vi "Main_Sigma_Single Scan_3.vi"() -> ()   [LabVIEW 2012]
uses:
  <vilib>/DAQmx/read.llb/DAQmx Read (Analog 1D DBL 1Chan NSamp).vi
  <vilib>/Instr/_visa.llb/VISA Configure Serial Port (Instr).vi
  <vilib>/DAQmx/create/channels.llb/DAQmx Create Channel (AI-Voltage-Basic).vi
  <vilib>/DAQmx/configure/timing.llb/DAQmx Timing (Sample Clock).vi
  <vilib>/DAQmx/configure/trigger.llb/DAQmx Start Trigger (Digital Edge).vi
  <vilib>/DAQmx/miscellaneous.llb/DAQmx Fill In Error Info.vi
  Global_data.vi
  <resource>/objmgr/daqmx.rc
  <vilib>/Platform/NI_3dgraph.lvlib
panel:
  out "Start. Pos.Y":dbl=18.8 format="%#.4f"
  out "숫자형 2":i32
  out "Start Pos. X":dbl=-22.5 format="%#.4f"
  out "숫자형":i32
  out "x < 0?":bool
  out "열거형":T1(ring)
  in  "Direction (+)":bool=TRUE
  out "No. X":i32=249
  out "No. Y":i32=13
  in  "X-length":dbl=5.0
  in  "Step X":dbl=0.02
  in  "COM Port":refnum<visa-resource-name>="COM1"
  in  "Baud Rate":u32=9600
  in  "Data bits":u16=8 min=5 max=8 step=1
  in  "stop bits":u16(ring)=10 items=["1.0"=10, "1.5"=15, "2.0"=20]
  in  "Parity":u16(ring) items=["None", "Odd", "Even", "Mark", "Space"]
  in  "1 Min":dbl=0.4
  in  "2 Max":dbl=4.0
  in  "1  Max":dbl=4.0
  in  "2 Min":dbl=0.4
  in  "Y-length":dbl=10.0
  in  "Step Y":dbl=0.1
  in  "1 Rate":dbl=0.2
  in  "2 Rate":dbl=0.4
  in  "Travel per Pulse (mm)":dbl=0.002
  in  "Cur. Pos X":dbl=-22.5 format="%#.4f"
  in  "Cur. Pos Y":dbl=18.8 format="%#.4f"
  in  "Save Speed":bool
  out "Move X":bool
  in  "Physical Channel":tag="Dev1/ai1"
  in  "Min Voltage":dbl=-0.2
  in  "Max Voltage":dbl=0.2
  in  "Terminal Configuration":i32(ring)=10083 items=["default"=-1, "RSE"=10083, "NRSE"=10078, "Differential"=10106, "Pseudodifferential"=12529]
  in  "rate":dbl=450000.0 format="%0.2f"
  in  "samples per channel":i32=100
  in  "3D Surface":refnum<k7>(container)
  in  "Stop Scan 3":bool
  in  "X-length count":dbl=20.0
  out "No.data":i32=3250
  in  "Save Scan mode":bool caption="Save Process"
  in  "Plot style":i32(ring)=5 items=["cwLine"=1, "cwPoint"=2, "cwLinePoint"=3, "cwHiddenLine"=4, "cwSurface"=5, "cwSurfaceLine"=6, "cwSurfaceNormal"=7, "cwContourLine"=8, "cwSurfaceContour"=9]
  in  "ViewMode":i32(ring) items=["cwViewXYPlane", "cwViewXZPlane", "cwViewYZPlane", "cwViewUserDefined"]
  in  "Emergency Stop":bool
  in  "Stop 3":bool
  in  "Home Y":bool
  in  "Home X":bool
  in  "Back":bool
  in  "Front":bool
  in  "Left":bool
  in  "Right":bool
  in  "Stop Scan":bool
  in  "Move Distance (mm)":dbl=5.0
  in  "Scan":bool
  in  "Open":bool
  in  "Edge":i32(ring)=10280 items=["Rising"=10280, "Falling"=10171]
  in  "Digital Trigger Source":tag="/Dev1/PFI8"
  # "Sensor  Channel"
  # "COM  Setting"
  # "Trigger Settings"
  # "Speed  Setting"
  # "Scan  Setting"
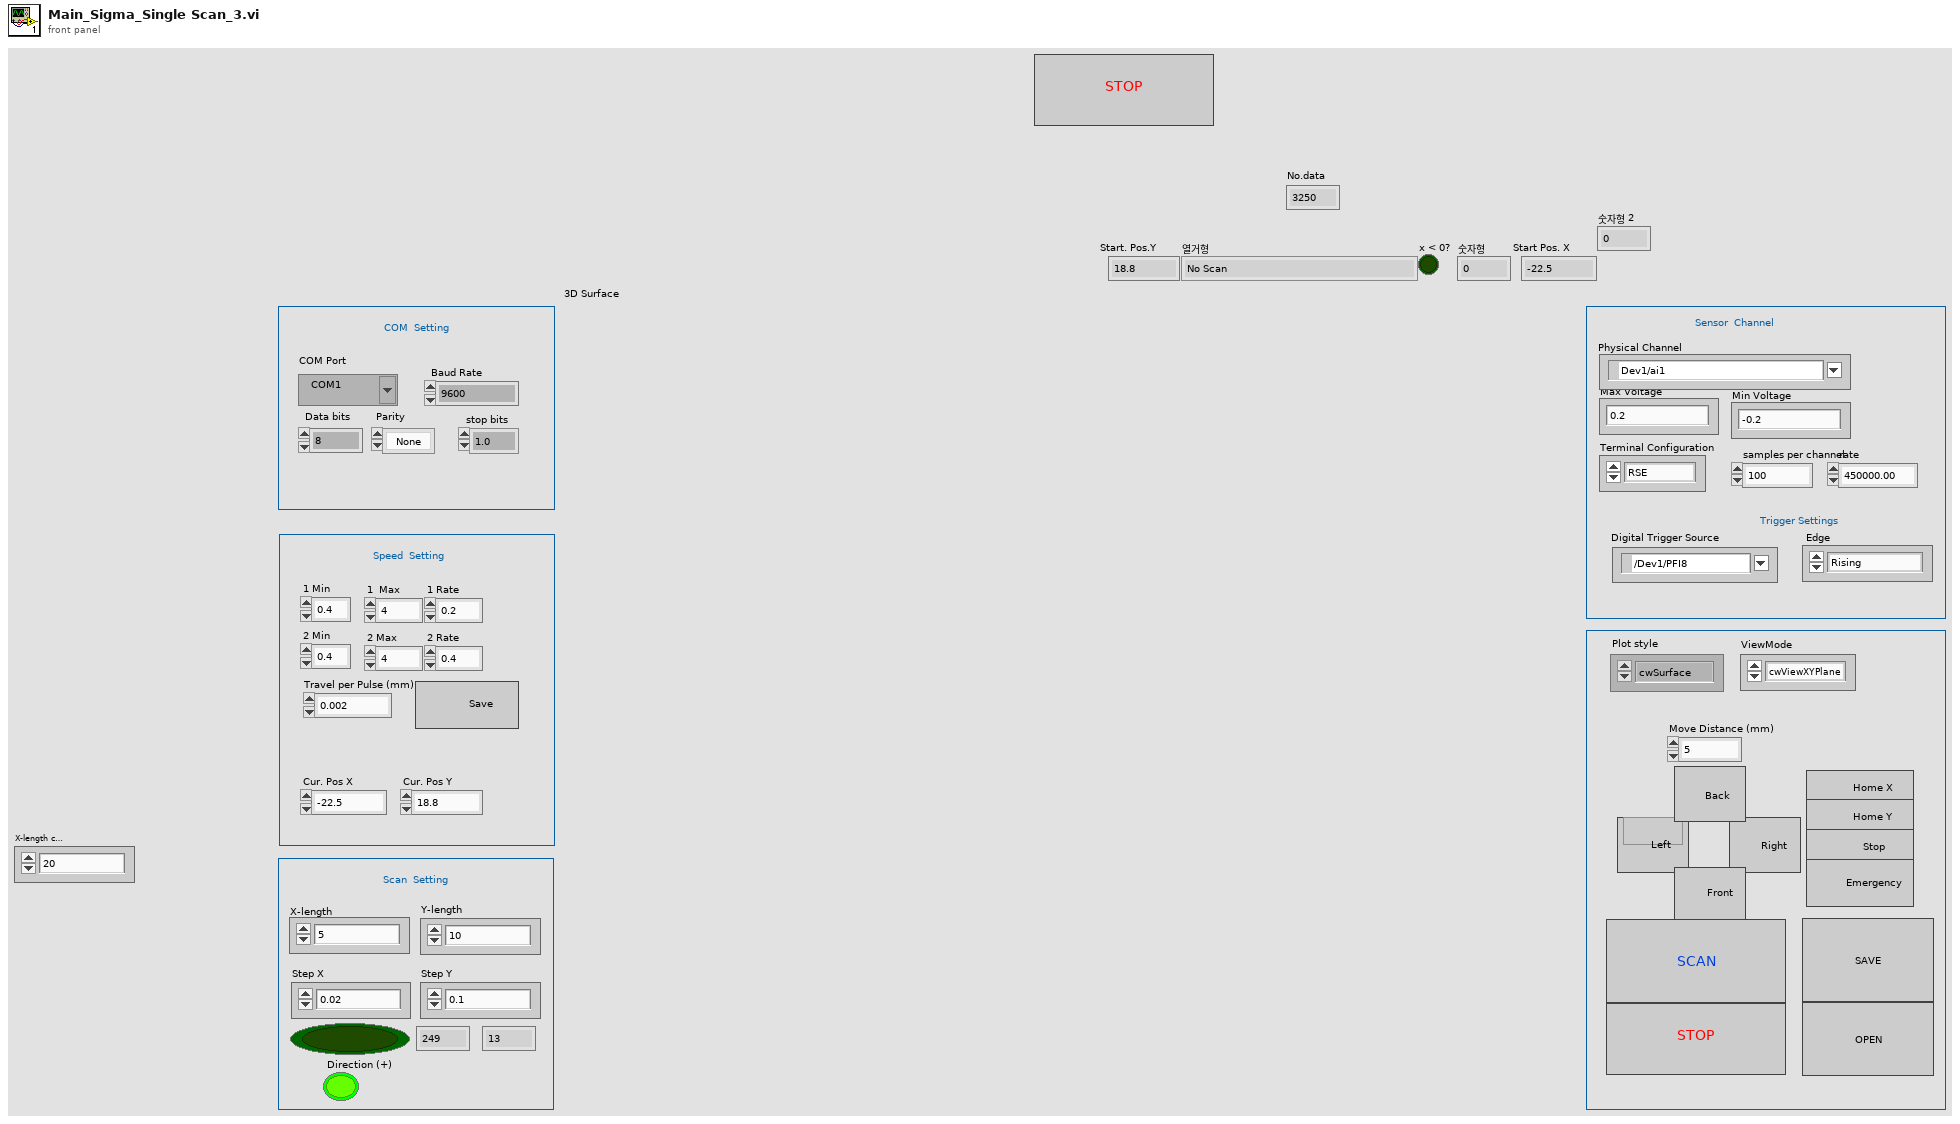
[diagram p1: front panel]
types:
  T1 = enum16{"No Scan", "Move X", "Wait to destination X", "Move Y", "Wait to destinatioin Y"}
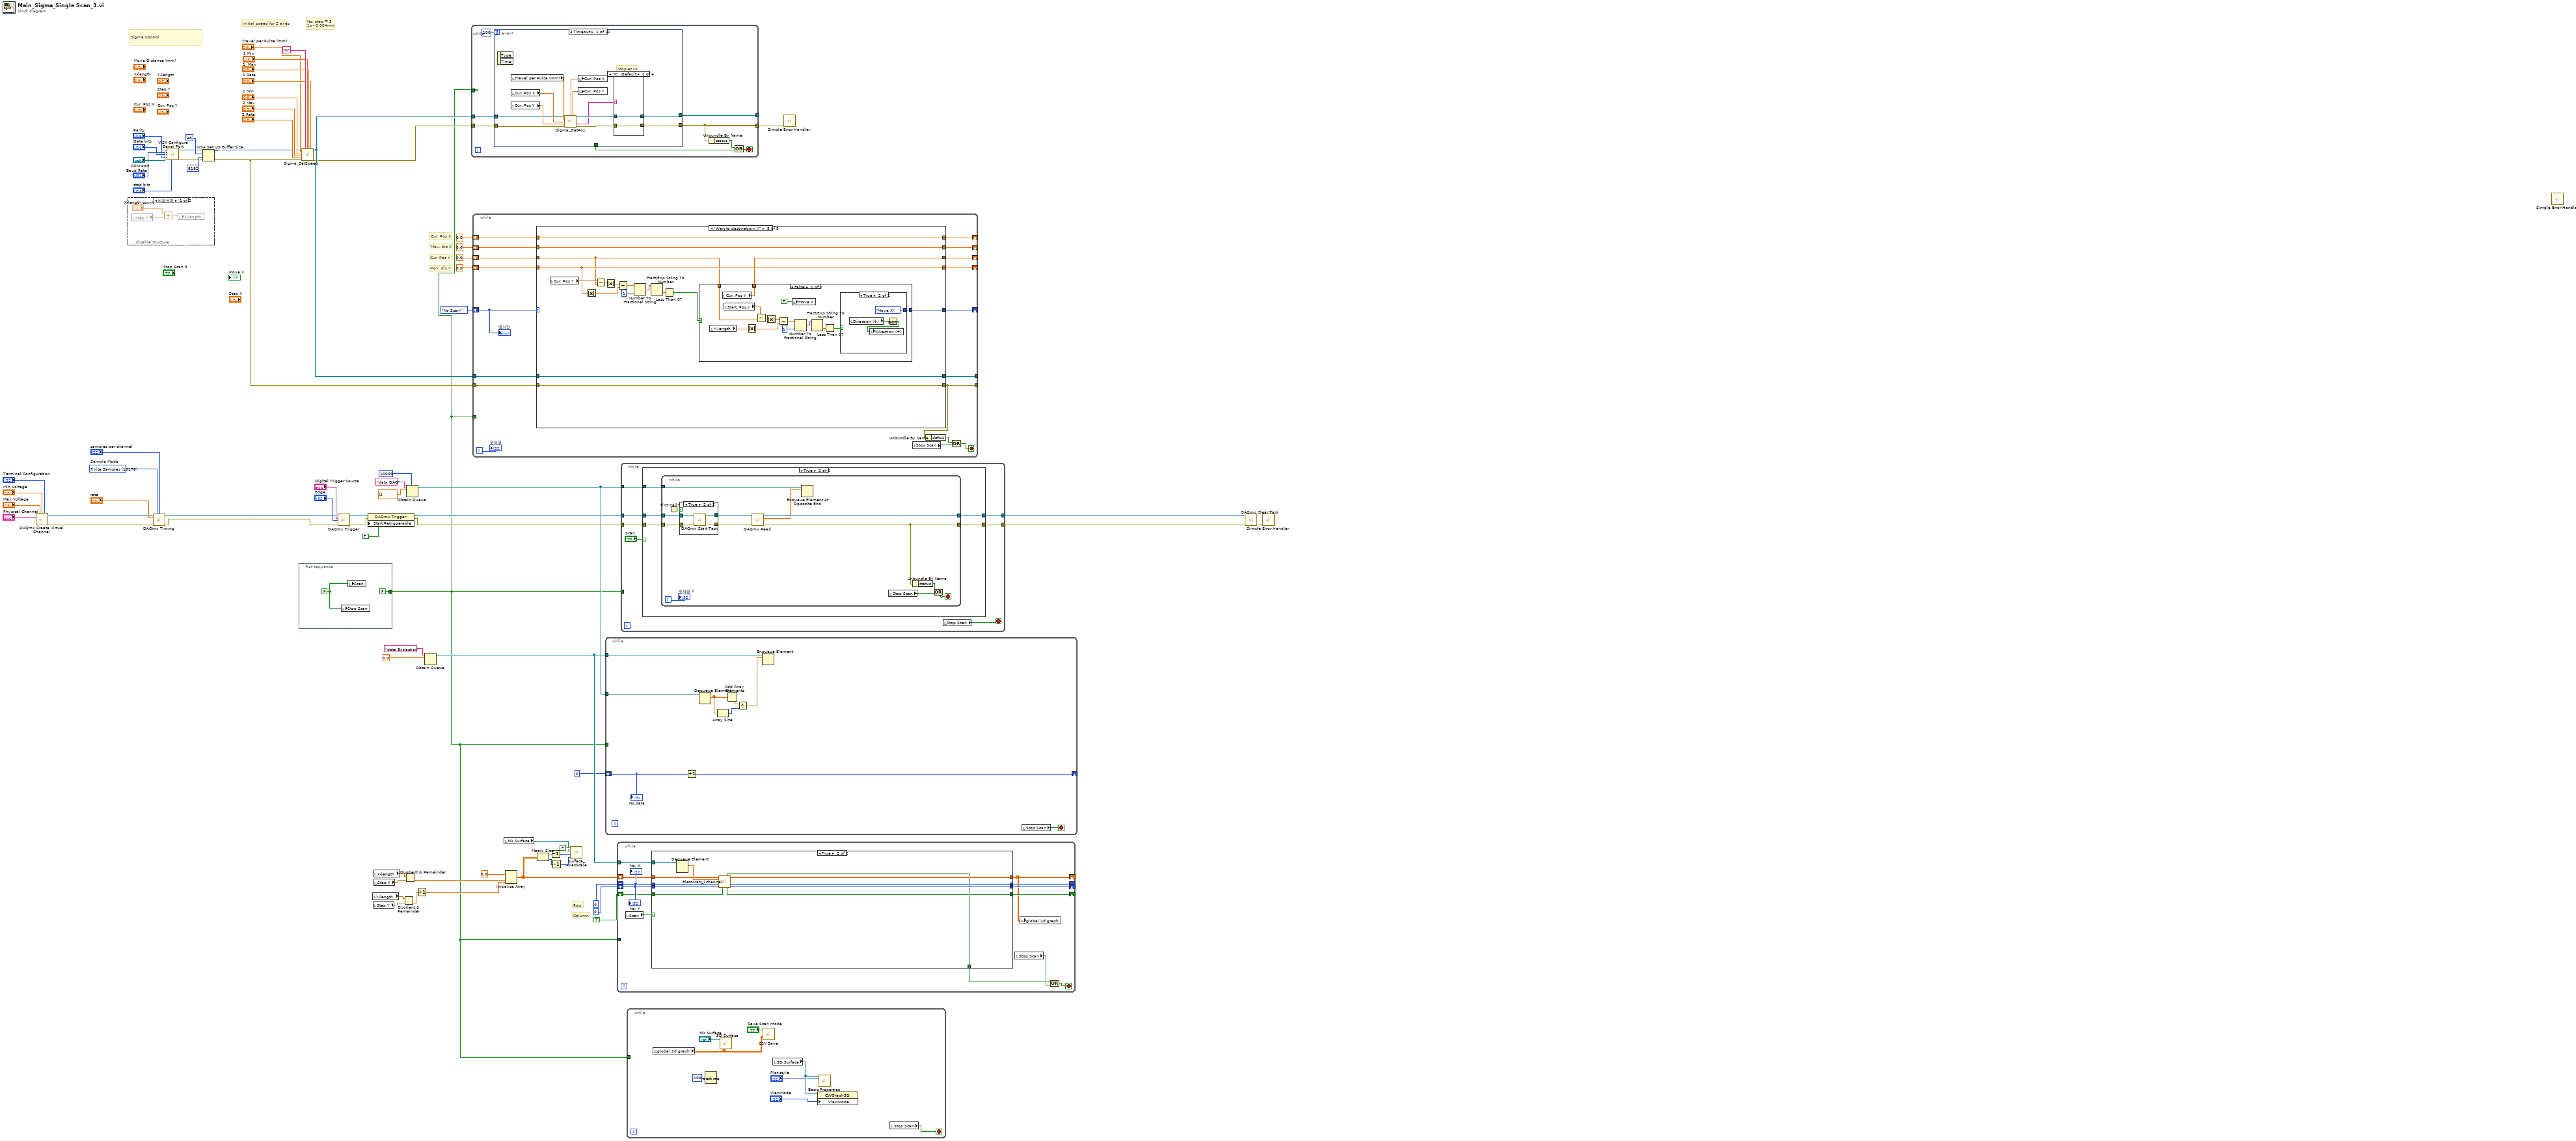
[diagram p0: block diagram]
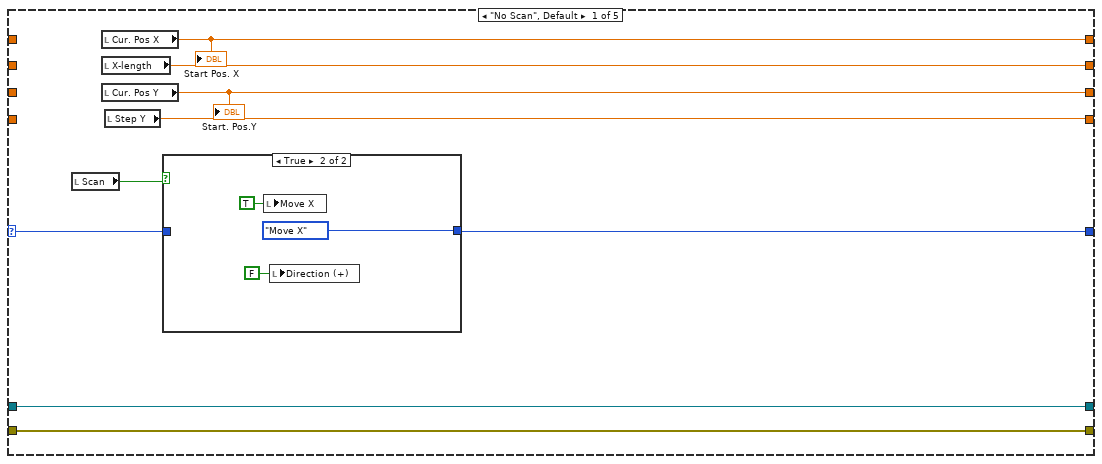
[diagram p2: hidden frame]
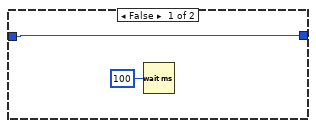
[diagram p3: hidden frame]
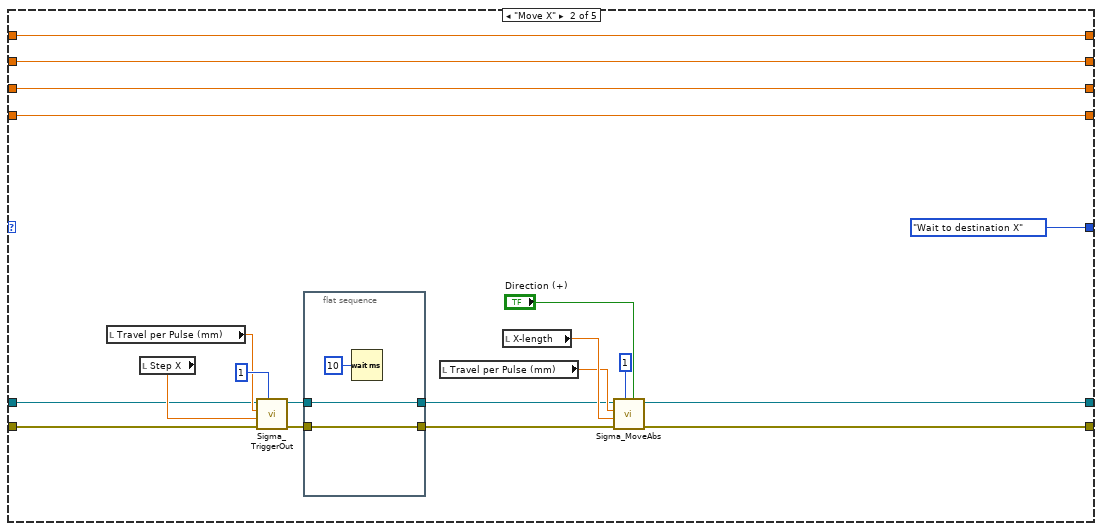
[diagram p4: hidden frame]
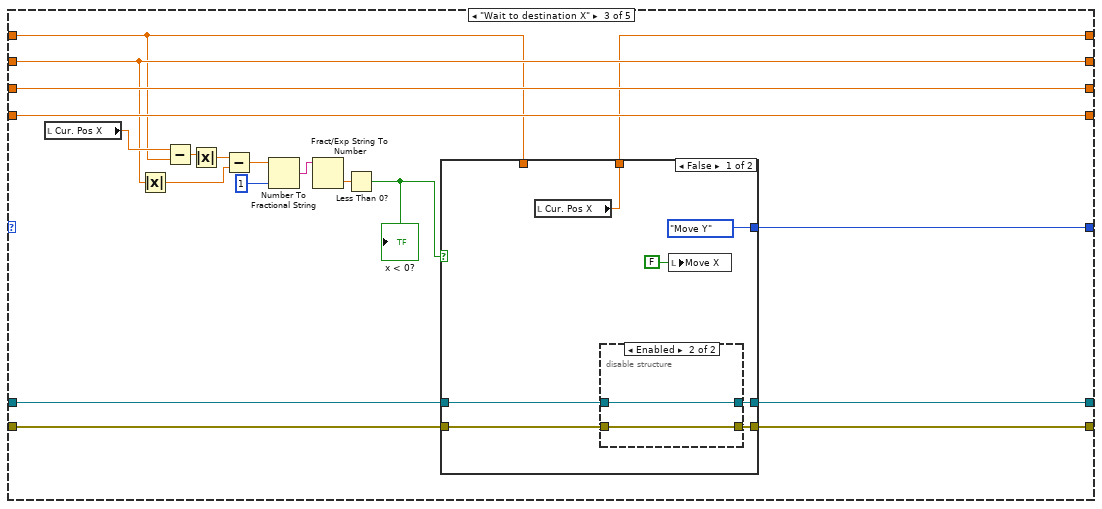
[diagram p5: hidden frame]
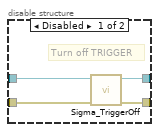
[diagram p6: hidden frame]
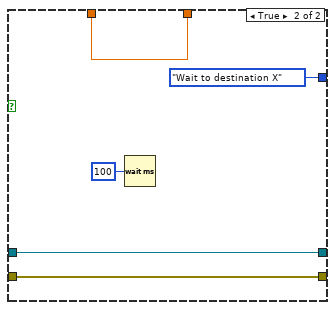
[diagram p7: hidden frame]
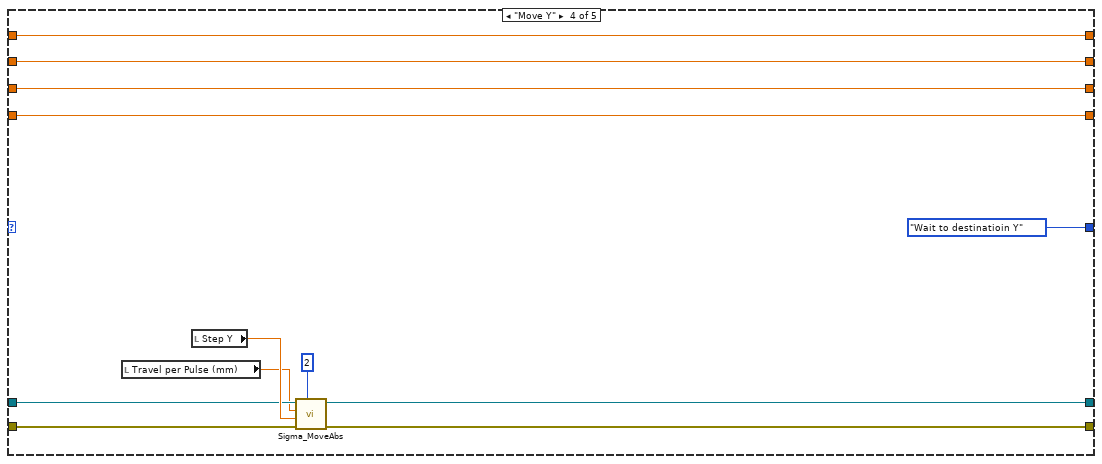
[diagram p8: hidden frame]
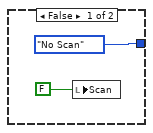
[diagram p9: hidden frame]
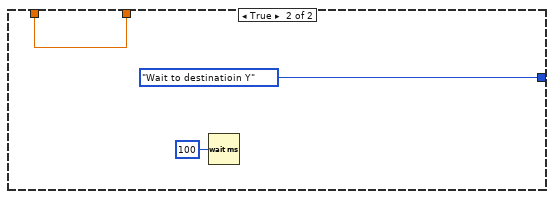
[diagram p10: hidden frame]
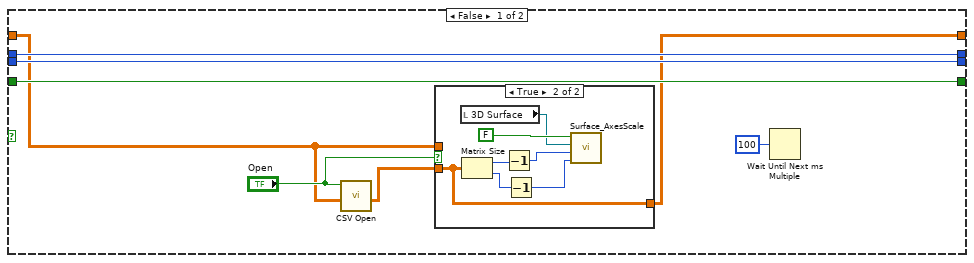
[diagram p11: hidden frame]
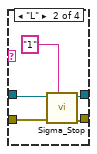
[diagram p16: hidden frame]
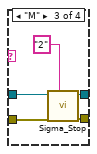
[diagram p17: hidden frame]
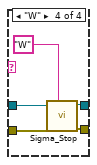
[diagram p18: hidden frame]
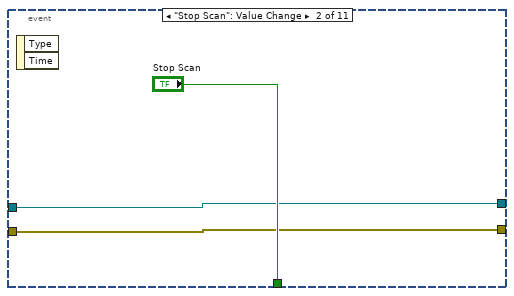
[diagram p19: hidden frame]
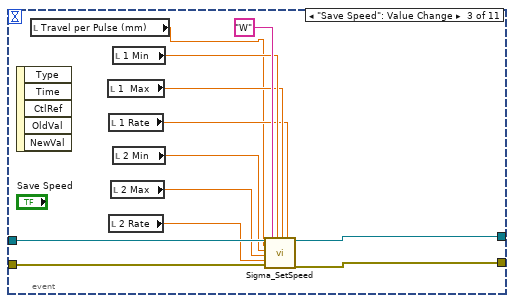
[diagram p20: hidden frame]
diagram:
  w46 = 10178 items=["Finite Samples"=10178, "Continuous Samples"=10123, "Hardware Timed Single Point"=12522]  # Sample Mode
  # "Mov. dis Y"
  # "Cur. Pos Y"
  # "Mov. dis X"
  # "Cur. Pos X"
  # "Column"
  # "Row"
  # "No. step = 5\n1p~0.004mm"
  # "Initial speed for 2 axes"
  # "Sigma Control"
  n1 = call-poly <vilib>:"DAQmx Create Virtual Channel.vi"("maximum value"="Max Voltage", "minimum value"="Min Voltage", "input terminal configuration"="Terminal Configuration", "physical channels"="Physical Channel") -> ("task out"=w54:refnum<k21>, "error out"=w55:errorcluster)  [unwired: 10 in]
  n2 = disable-structure shown="비활성화" {
    frame Disabled {
      n3 = local read "Step X"() -> (w78:dbl)
      n4 = Add(x="X-length count", y=w78) -> (x+y=w77:dbl)
      n5 = local write "X-length"(w77) -> ()
    }
    frame Enabled {
    }
  }
  n6 = call-poly <vilib>:"DAQmx Timing.vi"("task/channels in"=w54, "sample mode"=w46, "samples per channel"="samples per channel", "rate"="rate", "error in"=w55) -> ("task out"=w10:refnum<k21>, "error out"=w11:errorcluster)  [unwired: 9 in]
  n7 = call-poly "VISA Configure Serial Port"("VISA resource name"="COM Port", "baud rate (9600)"="Baud Rate", "data bits (8)"="Data bits", "parity (0:none)"="Parity", "stop bits (10: 1 bit)"="stop bits") -> ("VISA resource name out"=w62:refnum<visa-resource-name>, "error out"=w56:errorcluster)  [unwired: 9 in]
  n8 = VISA Set I/O Buffer Size(VISA resource name=w62, mask (16)=48, size (4096)=u32 8192, error in (no error)=w56) -> (VISA resource name out=w66:refnum<visa-resource-name>, error out=w65:errorcluster)
  n9 = flat-sequence {
    tunnel: [FALSE ("Scan")] -> w1
    frame #0 {
      w80 = FALSE ("Scan")
      n10 = local write "Stop Scan"(w80) -> ()
      n11 = local write "Scan"(w80) -> ()
    }
  }
  n12 = call "Sigma_SetSpeed.vi"("VISA resource name"=w66, "Travel per Pulse (0.004mm)"="Travel per Pulse (mm)", "Min (1mm) 2"="2 Min", "Max (2mm) 2"="2 Max", "Rate (1mm) 2"="2 Rate", "error in (no error)"=w65, "Axis (1)"="W", "Min (1mm)"="1 Min", "Max (2mm)"="1  Max", "Rate (1mm)"="1 Rate") -> ("VISA resource name out"=w3:refnum<visa-resource-name>, "error out"=w2:errorcluster)  [unwired: 8 in]
  n13 = call-poly <vilib>:"DAQmx Trigger.vi"("task/channels in"=w10, "source"="Digital Trigger Source", "edge"="Edge", "error in"=w11) -> ("task out"=w43:refnum<k21>, "error out"=w42:errorcluster)  [unwired: 10 in]
  n14 = property class="DAQmx Trigger"(reference=w43, error in=w42, "Start.Retriggerable"=TRUE) -> (reference out=w29:refnum<k21>, error out=w24:errorcluster)
  n15 = local read "Y-length"() -> (w32:dbl)
  n16 = local read "Step Y"() -> (w33:dbl)
  n17 = local read "X-length"() -> (w35:dbl)
  n18 = local read "Step X"() -> (w34:dbl)
  n19 = Quotient & Remainder(x=w32, y=w33) -> (floor(x/y)=w26:dbl)  [unwired: 1 out]
  n20 = Quotient & Remainder(x=w35, y=w34) -> (floor(x/y)=w28:dbl)  [unwired: 1 out]
  n21 = Obtain Queue(max queue size (-1, unlimited)=10000, name (unnamed)="data DAQ", element data type=dbl[] [] ("data")) -> (queue out=w40:refnum<queue>)  [unwired: 2 in, 2 out]
  n22 = Increment(x=w26) -> (x+1=w27:dbl)
  n23 = Obtain Queue(name (unnamed)="data Extraction", element data type=0.0) -> (queue out=w38:refnum<queue>)  [unwired: 3 in, 2 out]
  n24 = while {
    tunnel: w3 -> [w88]
    tunnel: [w83] -> _
    tunnel: w2 -> [w87]
    tunnel: [w85] -> w75
    tunnel: w1 -> [_]
    stop <- w84 stop-if-true
    n25 = event shown="[0] Timeout" {
      selector: _ -> [_ _ _ _ _ _ _ _ _ _ _]
      dyn-events: _ -> [_ _ _ _ _ _ _ _ _ _ _]
      timeout: 100 -> [_ _ _ _ _ _ _ _ _ _ _]
      tunnel: w88 -> [w94 w119 w132 w135 w150 w165 w180 w197 w209 w219 w231]
      tunnel: w87 -> [w93 w118 w129 w134 w149 w164 w179 w196 w208 w218 w230]
      tunnel: [w92 w119 w131 w137 w152 w167 w182 w194 w207 w221 w233] -> w83
      tunnel: [w91 w118 w130 w136 w151 w166 w181 w193 w206 w220 w232] -> w85
      tunnel: [_ "Stop Scan" _ _ _ _ _ _ _ _ _] -> w82
      event Timeout {
        # "Stop at LS"
        n26 = event-data() -> ()  [unwired: 1 in, 2 out]
        n27 = local read "Travel per Pulse (mm)"() -> (w96:dbl)
        n28 = local read "Cur. Pos X"() -> (w90:dbl)
        n29 = local read "Cur. Pos Y"() -> (w89:dbl)
        n30 = call "Sigma_GetPos.vi"("VISA resource name"=w94, "Travel per Pulse (mm)"=w96, "Init Pos X (mm)"=w90, "Init  Pos Y (mm)"=w89, "error in (no error)"=w93) -> ("Pos X (mm)"=w99:dbl, "Pos Y (mm)"=w100:dbl, "VISA resource name out"=w97:refnum<visa-resource-name>, "State String"=w95:string, "error out"=w98:errorcluster)  [unwired: 6 in]
        n31 = local write "Cur. Pos X"(w99) -> ()
        n32 = local write "Cur. Pos Y"(w100) -> ()
        n33 = case shown="\"K\", Default" w95 {
          tunnel: [w102 w107 w112 w117] -> w92
          tunnel: [w101 w106 w111 w116] -> w91
          tunnel: w97 -> [w102 w104 w109 w114]
          tunnel: w98 -> [w101 w103 w108 w113]
          frame "K", Default {
          }
          frame "L" {
            n34 = call "Sigma_Stop.vi"("Axis (1)"="1", "error in (no error)"=w103, "VISA resource name"=w104) -> ("error out"=w106:errorcluster, "VISA resource name out"=w107:refnum<visa-resource-name>)  [unwired: 7 in]
          }
          frame "M" {
            n35 = call "Sigma_Stop.vi"("Axis (1)"="2", "error in (no error)"=w108, "VISA resource name"=w109) -> ("error out"=w111:errorcluster, "VISA resource name out"=w112:refnum<visa-resource-name>)  [unwired: 7 in]
          }
          frame "W" {
            n36 = call "Sigma_Stop.vi"("Axis (1)"="W", "error in (no error)"=w113, "VISA resource name"=w114) -> ("error out"=w116:errorcluster, "VISA resource name out"=w117:refnum<visa-resource-name>)  [unwired: 7 in]
          }
        }
      }
      event "Stop Scan": Value Change {
        n37 = event-data() -> ()  [unwired: 1 in, 2 out]
      }
      event "Save Speed": Value Change {
        n38 = event-data() -> ()  [unwired: 1 in, 5 out]
        n39 = local read "Travel per Pulse (mm)"() -> (w121:dbl)
        n40 = local read "1  Max"() -> (w126:dbl)
        n41 = local read "1 Rate"() -> (w125:dbl)
        n42 = local read "2 Rate"() -> (w122:dbl)
        n43 = local read "2 Max"() -> (w123:dbl)
        n44 = local read "1 Min"() -> (w127:dbl)
        n45 = local read "2 Min"() -> (w124:dbl)
        n46 = call "Sigma_SetSpeed.vi"("VISA resource name"=w132, "Travel per Pulse (0.004mm)"=w121, "Min (1mm) 2"=w124, "Max (2mm) 2"=w123, "Rate (1mm) 2"=w122, "error in (no error)"=w129, "Axis (1)"="W", "Min (1mm)"=w127, "Max (2mm)"=w126, "Rate (1mm)"=w125) -> ("VISA resource name out"=w131:refnum<visa-resource-name>, "error out"=w130:errorcluster)  [unwired: 8 in]
      }
      event "Right": Value Change {
        n47 = event-data() -> ()  [unwired: 1 in, 1 out]
        n48 = case shown="True" "Right" {
          tunnel: [w139 w145] -> w137
          tunnel: [w138 w144] -> w136
          tunnel: w135 -> [w139 w147]
          tunnel: w134 -> [w138 w146]
          frame False {
          }
          frame True {
            n49 = local read "Travel per Pulse (mm)"() -> (w141:dbl)
            n50 = local read "Move Distance (mm)"() -> (w140:dbl)
            n51 = call "Sigma_MoveAbs.vi"("Direction (+)"=FALSE, "Axis (1)"=1, "error in (no error)"=w146, "Travel (1mm)"=w140, "Travel per Pulse (0.004mm)"=w141, "VISA resource name"=w147) -> ("error out"=w144:errorcluster, "VISA resource name out"=w145:refnum<visa-resource-name>)  [unwired: 4 in]
          }
        }
      }
      event "Left": Value Change {
        n52 = event-data() -> ()  [unwired: 1 in, 1 out]
        n53 = case shown="True" "Left" {
          tunnel: [w154 w161] -> w152
          tunnel: [w153 w160] -> w151
          tunnel: w150 -> [w154 w162]
          tunnel: w149 -> [w153 w159]
          frame False {
          }
          frame True {
            n54 = local read "Travel per Pulse (mm)"() -> (w156:dbl)
            n55 = local read "Move Distance (mm)"() -> (w155:dbl)
            n56 = call "Sigma_MoveAbs.vi"("Direction (+)"=TRUE, "Axis (1)"=1, "error in (no error)"=w159, "Travel (1mm)"=w155, "Travel per Pulse (0.004mm)"=w156, "VISA resource name"=w162) -> ("error out"=w160:errorcluster, "VISA resource name out"=w161:refnum<visa-resource-name>)  [unwired: 4 in]
          }
        }
      }
      event "Front": Value Change {
        n57 = event-data() -> ()  [unwired: 1 in, 1 out]
        n58 = case shown="True" "Front" {
          tunnel: [w169 w175] -> w167
          tunnel: [w168 w174] -> w166
          tunnel: w165 -> [w169 w177]
          tunnel: w164 -> [w168 w176]
          frame False {
          }
          frame True {
            n59 = local read "Travel per Pulse (mm)"() -> (w171:dbl)
            n60 = local read "Move Distance (mm)"() -> (w170:dbl)
            n61 = call "Sigma_MoveAbs.vi"("Direction (+)"=FALSE, "Axis (1)"=2, "error in (no error)"=w176, "Travel (1mm)"=w170, "Travel per Pulse (0.004mm)"=w171, "VISA resource name"=w177) -> ("error out"=w174:errorcluster, "VISA resource name out"=w175:refnum<visa-resource-name>)  [unwired: 4 in]
          }
        }
      }
      event "Back": Value Change {
        n62 = event-data() -> ()  [unwired: 1 in, 1 out]
        n63 = case shown="True" "Back" {
          tunnel: [w184 w190] -> w182
          tunnel: [w183 w189] -> w181
          tunnel: w180 -> [w184 w192]
          tunnel: w179 -> [w183 w191]
          frame False {
          }
          frame True {
            n64 = local read "Travel per Pulse (mm)"() -> (w186:dbl)
            n65 = local read "Move Distance (mm)"() -> (w185:dbl)
            n66 = call "Sigma_MoveAbs.vi"("Direction (+)"=TRUE, "Axis (1)"=2, "error in (no error)"=w191, "Travel (1mm)"=w185, "Travel per Pulse (0.004mm)"=w186, "VISA resource name"=w192) -> ("error out"=w189:errorcluster, "VISA resource name out"=w190:refnum<visa-resource-name>)  [unwired: 4 in]
          }
        }
      }
      event "Home X": Value Change {
        n67 = event-data() -> ()  [unwired: 1 in, 1 out]
        n68 = case shown="True" "Home X" {
          tunnel: [w199 w202] -> w194
          tunnel: [w198 w201] -> w193
          tunnel: w197 -> [w199 w204]
          tunnel: w196 -> [w198 w203]
          frame False {
          }
          frame True {
            n69 = call "Sigma_Home.vi"("Axis (1)"="1", "error in (no error)"=w203, "VISA resource name"=w204) -> ("error out"=w201:errorcluster, "VISA resource name out"=w202:refnum<visa-resource-name>)  [unwired: 7 in]
          }
        }
      }
      event "Home Y": Value Change {
        n70 = event-data() -> ()  [unwired: 1 in, 1 out]
        n71 = case shown="True" "Home Y" {
          tunnel: [w211 w214] -> w207
          tunnel: [w210 w213] -> w206
          tunnel: w209 -> [w211 w216]
          tunnel: w208 -> [w210 w215]
          frame False {
          }
          frame True {
            n72 = call "Sigma_Home.vi"("Axis (1)"="2", "error in (no error)"=w215, "VISA resource name"=w216) -> ("error out"=w213:errorcluster, "VISA resource name out"=w214:refnum<visa-resource-name>)  [unwired: 7 in]
          }
        }
      }
      event "Stop 3": Value Change {
        n73 = event-data() -> ()  [unwired: 1 in, 1 out]
        n74 = case shown="True" "Stop 3" {
          tunnel: [w223 w224] -> w221
          tunnel: [w222 w225] -> w220
          tunnel: w219 -> [w223 w227]
          tunnel: w218 -> [w222 w226]
          frame False {
          }
          frame True {
            n75 = call "Sigma_Stop.vi"("Axis (1)"="W", "error in (no error)"=w226, "VISA resource name"=w227) -> ("error out"=w225:errorcluster, "VISA resource name out"=w224:refnum<visa-resource-name>)  [unwired: 7 in]
          }
        }
      }
      event "Emergency Stop": Value Change {
        n76 = event-data() -> ()  [unwired: 1 in, 1 out]
        n77 = case shown="True" "Emergency Stop" {
          tunnel: [w235 w238] -> w233
          tunnel: [w234 w237] -> w232
          tunnel: w231 -> [w235 w240]
          tunnel: w230 -> [w234 w239]
          frame False {
          }
          frame True {
            n78 = call "Sigma_Stop.vi"("Axis (1)"="E", "error in (no error)"=w239, "VISA resource name"=w240) -> ("error out"=w237:errorcluster, "VISA resource name out"=w238:refnum<visa-resource-name>)  [unwired: 7 in]
          }
        }
      }
    }
    n79 = Unbundle By Name(w85) -> ("status"=w86:bool)
    n80 = Compound Arithmetic op=OR(w86, w82) -> (w84:bool)
  }
  n81 = while {
    shift-right: [w257] -> _
    shift-left: T1."No Scan" -> [w258]
    shift-right: [w253] -> _
    shift-left: 0.0 ("Current  Position (mm)") -> [w252]
    shift-right: [w251] -> _
    shift-left: 0.0 ("Current  Position (mm)") -> [w250]
    shift-right: [w249] -> _
    shift-left: 0.0 ("Current  Position (mm)") -> [w248]
    shift-right: [w247] -> _
    shift-left: 0.0 ("Current  Position (mm)") -> [w246]
    tunnel: w3 -> [w256]
    tunnel: [w254] -> _
    tunnel: w2 -> [w255]
    tunnel: [w242] -> _
    tunnel: w1 -> [_]
    i -> [w241]
    stop <- w243 stop-if-true
    n82 = case shown="\"Wait to destinatioin Y\"" w258 {
      selector: w258 -> [w265 _ _ _ _]
      tunnel: [w266 T1."Wait to destination X" w302 T1."Wait to destinatioin Y" w350] -> w257
      tunnel: w256 -> [w260 w279 w301 w342 w349]
      tunnel: w255 -> [w259 w278 w300 w341 w348]
      tunnel: [w260 w288 w299 w338 w349] -> w254
      tunnel: [w259 w287 w298 w337 w348] -> w242
      tunnel: [w264 w286 w297 w336 w354] -> w253
      tunnel: w252 -> [_ w286 w296 w336 w354]
      tunnel: [w263 w285 w304 w335 w352] -> w251
      tunnel: w250 -> [_ w285 w304 w335 w352]
      tunnel: [w262 w284 w307 w334 w347] -> w249
      tunnel: w248 -> [_ w284 w307 w334 w345]
      tunnel: [w261 w283 w306 w333 w346] -> w247
      tunnel: w246 -> [_ w283 w306 w333 w346]
      frame "No Scan", Default {
        n83 = local read "Scan"() -> (w267:bool)
        n84 = local read "Cur. Pos X"() -> (w264:dbl)
        "Start Pos. X" <- w264
        n85 = local read "X-length"() -> (w263:dbl)
        n86 = local read "Cur. Pos Y"() -> (w262:dbl)
        "Start. Pos.Y" <- w262
        n87 = local read "Step Y"() -> (w261:dbl)
        n88 = case shown="True" w267 {
          tunnel: [w269 T1."Move X"] -> w266
          tunnel: w265 -> [w269 _]
          frame False {
            n89 = Wait (ms)(milliseconds to wait=u32 100) -> ()  [unwired: 1 out]
          }
          frame True {
            n90 = local write "Move X"(TRUE ("Move X")) -> ()
            n91 = local write "Direction (+)"(FALSE ("Direction (+)")) -> ()
          }
        }
      }
      frame "Move X" {
        n92 = local read "Travel per Pulse (mm)"() -> (w280:dbl)
        n93 = local read "Step X"() -> (w281:dbl)
        n94 = call "Sigma_TriggerOut.vi"("Axis(1)"=1, "error in (no error)"=w278, "Trigger distance (mm)"=w281, "Travel per Pulse (mm)"=w280, "VISA resource name"=w279) -> ("error out"=w274:errorcluster, "VISA resource name out"=w276:refnum<visa-resource-name>)  [unwired: 5 in]
        n95 = flat-sequence {
          tunnel: [w295] -> w277
          tunnel: w276 -> [w295]
          tunnel: [w294] -> w275
          tunnel: w274 -> [w294]
          frame #0 {
            n96 = Wait (ms)(milliseconds to wait=u32 10) -> ()  [unwired: 1 out]
          }
        }
        n97 = local read "Travel per Pulse (mm)"() -> (w290:dbl)
        n98 = local read "X-length"() -> (w291:dbl)
        n99 = call "Sigma_MoveAbs.vi"("Direction (+)"="Direction (+)", "Axis (1)"=1, "error in (no error)"=w275, "Travel (1mm)"=w291, "Travel per Pulse (0.004mm)"=w290, "VISA resource name"=w277) -> ("error out"=w287:errorcluster, "VISA resource name out"=w288:refnum<visa-resource-name>)  [unwired: 4 in]
      }
      frame "Wait to destination X" {
        n100 = local read "Cur. Pos X"() -> (w305:dbl)
        n101 = Absolute Value(x=w304) -> (abs(x)=w310:dbl)
        n102 = Subtract(x=w305, y=w296) -> (x-y=w314:dbl)
        n103 = Absolute Value(x=w314) -> (abs(x)=w311:dbl)
        n104 = Subtract(x=w311, y=w310) -> (x-y=w308:dbl)
        n105 = Number To Fractional String(number=w308, precision (6)=i16 1 ("정밀도(6)")) -> (F-format string=w313:string)  [unwired: 2 in]
        n106 = Fract/Exp String To Number(string=w313) -> (number=w309:dbl)  [unwired: 3 in, 1 out]
        n107 = Less Than 0?(x=w309) -> (x < 0?=w303:bool)
        "x < 0?" <- w303
        n108 = case shown="False" w303 {
          tunnel: [T1."Move Y" T1."Wait to destination X"] -> w302
          tunnel: w301 -> [w319 w331]
          tunnel: w300 -> [w318 w330]
          tunnel: [w317 w331] -> w299
          tunnel: [w316 w330] -> w298
          tunnel: [w315 w328] -> w297
          tunnel: w296 -> [_ w328]
          frame False {
            n109 = local read "Cur. Pos X"() -> (w315:dbl)
            n110 = disable-structure shown="Enabled" {
              disable-tunnel: w319 -> [w325 w327]
              disable-tunnel: w318 -> [w324 w326]
              disable-tunnel: [w323 w327] -> w317
              disable-tunnel: [w322 w326] -> w316
              frame Disabled {
                # "Turn off TRIGGER"
                n111 = call "Sigma_TriggerOff.vi"("error in (no error)"=w324, "VISA resource name"=w325) -> ("error out"=w322:errorcluster, "VISA resource name out"=w323:refnum<visa-resource-name>)  [unwired: 8 in]
              }
              frame Enabled {
              }
            }
            n112 = local write "Move X"(FALSE ("Move X")) -> ()
          }
          frame True {
            n113 = Wait (ms)(milliseconds to wait=u32 100) -> ()  [unwired: 1 out]
          }
        }
      }
      frame "Move Y" {
        n114 = local read "Travel per Pulse (mm)"() -> (w340:dbl)
        n115 = local read "Step Y"() -> (w343:dbl)
        n116 = call "Sigma_MoveAbs.vi"("Axis (1)"=2, "error in (no error)"=w341, "Travel (1mm)"=w343, "Travel per Pulse (0.004mm)"=w340, "VISA resource name"=w342) -> ("error out"=w337:errorcluster, "VISA resource name out"=w338:refnum<visa-resource-name>)  [unwired: 5 in]
      }
      frame "Wait to destinatioin Y" {
        n117 = local read "Cur. Pos Y"() -> (w353:dbl)
        n118 = Absolute Value(x=w346) -> (abs(x)=w357:dbl)
        n119 = Subtract(x=w353, y=w345) -> (x-y=w361:dbl)
        n120 = Absolute Value(x=w361) -> (abs(x)=w358:dbl)
        n121 = Subtract(x=w358, y=w357) -> (x-y=w355:dbl)
        n122 = Number To Fractional String(number=w355, precision (6)=i16 1 ("정밀도(6)")) -> (F-format string=w360:string)  [unwired: 2 in]
        n123 = Fract/Exp String To Number(string=w360) -> (number=w356:dbl)  [unwired: 3 in, 1 out]
        n124 = Less Than 0?(x=w356) -> (x < 0?=w351:bool)
        n125 = case shown="False" w351 {
          tunnel: [w375 T1."Wait to destinatioin Y"] -> w350
          tunnel: w345 -> [w366 w381]
          tunnel: [w363 w381] -> w347
          frame False {
            n126 = local read "Y-length"() -> (w367:dbl)
            n127 = local read "Cur. Pos Y"() -> (w363:dbl)
            n128 = local read "Start. Pos.Y"() -> (w362:dbl)
            n129 = Absolute Value(x=w367) -> (abs(x)=w370:dbl)
            n130 = Subtract(x=w362, y=w366) -> (x-y=w374:dbl)
            n131 = Absolute Value(x=w374) -> (abs(x)=w371:dbl)
            n132 = Subtract(x=w371, y=w370) -> (x-y=w368:dbl)
            n133 = local write "Move X"(FALSE ("Move X")) -> ()
            n134 = Number To Fractional String(number=w368, precision (6)=i16 1 ("정밀도(6)")) -> (F-format string=w373:string)  [unwired: 2 in]
            n135 = Fract/Exp String To Number(string=w373) -> (number=w369:dbl)  [unwired: 3 in, 1 out]
            n136 = Less Than 0?(x=w369) -> (x < 0?=w364:bool)
            n137 = case shown="True" w364 {
              tunnel: [T1."No Scan" T1."Move X"] -> w375
              frame False {
                n138 = local write "Scan"(FALSE ("Move X")) -> ()
              }
              frame True {
                n139 = local read "Direction (+)"() -> (w379:bool)
                n140 = Not(x=w379) -> (.not. x?=w378:bool)
                n141 = local write "Direction (+)"(w378) -> ()
              }
            }
          }
          frame True {
            n142 = Wait (ms)(milliseconds to wait=u32 100) -> ()  [unwired: 1 out]
          }
        }
      }
    }
    n143 = local read "Stop Scan"() -> (w244:bool)
    n144 = Unbundle By Name(w242) -> ("status"=w245:bool)
    n145 = Compound Arithmetic op=OR(w245, w244) -> (w243:bool)
    "열거형" <- w258
    "숫자형" <- w241
  }
  n146 = local read "3D Surface"() -> (w12:refnum<k7>)
  n147 = Initialize Array(0.0 ("element"), w28, w27) -> (w17:dbl[][])
  n148 = Matrix Size(0:w17) -> (1:w18:i32, 2:w19:i32)
  n149 = Decrement(x=w18) -> (x-1=w22:i32)
  n150 = Decrement(x=w19) -> (x-1=w21:i32)
  n151 = call "Surface_AxesScale.vi"("Y-axis Max"=w21, "X-axis max"=w22, "3D Surface"=w12, "Auto Scale"=FALSE) -> ()  [unwired: 8 in]
  n152 = while {
    tunnel: w40 -> [w392]
    tunnel: w38 -> [w391]
    shift-right: [w389] -> _
    shift-left: 0 -> [w390]
    tunnel: w1 -> [_]
    stop <- w388 stop-if-true
    n153 = Increment(x=w390) -> (x+1=w389:i32)
    n154 = Dequeue Element(queue=w392) -> (element=w387:dbl[])  [unwired: 2 in, 3 out]
    n155 = Array Size(array=w387) -> (size(s)=w386:i32)
    n156 = Add Array Elements(numeric array=w387) -> (sum=w385:dbl)
    n157 = Divide(x=w385, y=w386) -> (x/y=w384:dbl)
    n158 = Enqueue Element(queue=w391, element=w384) -> ()  [unwired: 2 in, 3 out]
    n159 = local read "Stop Scan"() -> (w388:bool)
    "No.data" <- w390
  }
  n160 = while {
    shift-right: [w403] -> _
    shift-left: 0 -> [w405]
    shift-right: [w402] -> _
    shift-left: 0 -> [w404]
    tunnel: w38 -> [w401]
    shift-right: [w393] -> _
    shift-left: w17 -> [w400]
    shift-right: [w394] -> _
    shift-left: TRUE ("Output Direction") -> [w395]
    tunnel: w1 -> [_]
    stop <- w397 stop-if-true
    n161 = local read "Scan"() -> (w399:bool)
    n162 = case shown="True" w399 {
      tunnel: w405 -> [w413 w432]
      tunnel: w404 -> [w412 w431]
      tunnel: [w413 w430] -> w403
      tunnel: [w412 w429] -> w402
      tunnel: w401 -> [_ w428]
      tunnel: w400 -> [w407 w426]
      tunnel: [w406 w422] -> w393
      tunnel: [_ w425] -> w396
      tunnel: w395 -> [w411 w424]
      tunnel: [w411 w423] -> w394
      frame False {
        n163 = call "CSV Open.vi"("2D Array In"=w407, "Open"="Open") -> ("2D Array Out"=w410:dbl[][])  [unwired: 9 in]
        n164 = case shown="True" "Open" {
          tunnel: w410 -> [_ w416]
          tunnel: [w414 w416] -> w406
          tunnel: w407 -> [w414 _]
          frame False {
          }
          frame True {
            n165 = local read "3D Surface"() -> (w415:refnum<k7>)
            n166 = Matrix Size(0:w416) -> (1:w417:i32, 2:w418:i32)
            n167 = Decrement(x=w417) -> (x-1=w421:i32)
            n168 = Decrement(x=w418) -> (x-1=w420:i32)
            n169 = call "Surface_AxesScale.vi"("Y-axis Max"=w420, "X-axis max"=w421, "3D Surface"=w415, "Auto Scale"=FALSE) -> ()  [unwired: 8 in]
          }
        }
        n170 = Wait Until Next ms Multiple(millisecond multiple=u32 100 ("ms 배수")) -> ()  [unwired: 1 out]
      }
      frame True {
        n171 = Dequeue Element(queue=w428) -> (element=w427:dbl)  [unwired: 2 in, 3 out]
        n172 = call "EletoMatr_1channel.vi"("Input Array X"=w426, "Input data"=w427, "In Row"=w432, "In Column"=w431, "Input Direction"=w424) -> ("Completed"=w425:bool, "Out Array X"=w422:dbl[][], "Out Row"=w430:i32, "Output Direction"=w423:bool, "Out Column"=w429:i32)  [unwired: 6 in]
      }
    }
    n173 = local read "Stop Scan"() -> (w398:bool)
    n174 = global write "Global_data.vi" "global 2d graph"(w393) -> ()
    n175 = Compound Arithmetic op=OR(w396, w398) -> (w397:bool)
    "No. Y" <- w404
    "No. X" <- w405
  }
  n176 = while {
    tunnel: w29 -> [w439]
    tunnel: [w438] -> w48
    tunnel: [w437] -> w47
    tunnel: w24 -> [w436]
    tunnel: w40 -> [w435]
    tunnel: w1 -> [_]
    stop <- w434 stop-if-true
    n177 = case shown="True" "Scan" {
      tunnel: w439 -> [w441 w446]
      tunnel: [w441 w445] -> w438
      tunnel: [w440 w444] -> w437
      tunnel: w436 -> [w440 w443]
      tunnel: w435 -> [_ w442]
      frame False {
      }
      frame True {
        n178 = while {
          tunnel: w446 -> [w453]
          tunnel: [w459] -> w445
          tunnel: [w458] -> w444
          tunnel: w443 -> [w452]
          tunnel: w442 -> [w457]
          i -> [w447]
          stop <- w455 stop-if-true
          n179 = First Call?() -> (First Call?: T/F=w449:bool)
          n180 = case shown="True" w449 {
            tunnel: w453 -> [w460 w465]
            tunnel: w452 -> [w461 w464]
            tunnel: [w460 w463] -> w451
            tunnel: [w461 w462] -> w450
            frame False {
            }
            frame True {
              n181 = call <vilib>:"DAQmx Start Task.vi"("task/channels in"=w465, "error in"=w464) -> ("task out"=w463:refnum<k21>, "error out"=w462:errorcluster)  [unwired: 12 in]
            }
          }
          n182 = call-poly <vilib>:"DAQmx Read.vi"("task/channels in"=w451, "error in"=w450) -> ("task out"=w459:refnum<k21>, "data"=w448:dbl[], "error out"=w458:errorcluster)  [unwired: 11 in]
          n183 = Enqueue Element At Opposite End(queue=w457, element=w448) -> ()  [unwired: 2 in, 3 out]
          n184 = local read "Stop Scan"() -> (w454:bool)
          n185 = Unbundle By Name(w458) -> ("status"=w456:bool)
          n186 = Or(x=w456, y=w454) -> (x .or. y?=w455:bool)
          "숫자형 2" <- w447
        }
      }
    }
    n187 = local read "Stop Scan"() -> (w434:bool)
  }
  n188 = while {
    tunnel: w1 -> [_]
    stop <- w471 stop-if-true
    n189 = global read "Global_data.vi" "global 2d graph"() -> (w466:dbl[][])
    n190 = Wait (ms)(milliseconds to wait=u32 100) -> ()  [unwired: 1 out]
    n191 = call <vilib>:"3D Surface.vi"("z matrix"=w466, "3D graph"="3D Surface") -> ()  [unwired: 8 in, 2 out]
    n192 = call "CSV Save.vi"("Array"=w466, "Save Button"="Save Scan mode") -> ()  [unwired: 9 in, 1 out]
    n193 = local read "3D Surface"() -> (w473:refnum<k7>)
    n194 = property class="CWGraph3D"(reference=w473, "ViewMode"="ViewMode") -> ()  [unwired: 1 in, 2 out]
    n195 = call <vilib>:"Basic Properties.vi"("3D graph"=w473, "plot style"="Plot style") -> ()  [unwired: 12 in, 2 out]
    n196 = local read "Stop Scan"() -> (w471:bool)
  }
  n197 = call <vilib>:"Simple Error Handler.vi"("error in (no error)"=w75) -> ()  [unwired: 4 in, 5 out]
  n198 = call <vilib>:"DAQmx Clear Task.vi"("task in"=w48, "error in"=w47) -> ("error out"=w53:errorcluster)  [unwired: 13 in]
  n199 = call <vilib>:"Simple Error Handler.vi"("error in (no error)"=w53) -> ()  [unwired: 4 in, 5 out]
  n200 = call <vilib>:"Simple Error Handler.vi"() -> ()  [unwired: 5 in, 5 out]
